vi "FTW_AppLauncher-Core_Initialize.vi"(0 "Initialization Sequence":string, 5 "FTW Actor Instance Configuration":string, 11 "error in (no error)":errorcluster) -> (4 "Actor Template-Core out":refnum<class "FTW-AppLauncher-Core.lvclass">, 6 "Event Refnums":T1, 10 "Refresh Period":dbl, 15 "error out":errorcluster)   [LabVIEW 2015, in "FTW-AppLauncher-Core.lvclass"]
uses:
  FTW-AppLauncher-Core.lvclass
  source/actor/Message/Request/FTW-Message-IncomingRequest.lvclass
  source/actor/Message/Base/FTW-Message.lvclass
  FTW-AppLauncher-Core.lvclass/FTW-AppLauncher-Core.ctl
  source/actor/Instance/FTW-ActorInstance.lvclass/FTW-ActorInstance.ctl
  source/Error/FTW-ERR-NoErrorConstant.vi
  source/JSON/FTW-JSON-Core-LibraryFilepath.vi
  source/Error/FTW-ERR-ThrowError.vi
  source/JSON/core/FTW-JSON-Core-EncodingFlags.vi
  source/Reflection/FTW-Reflection-Type.vi
  source/CodeGen/JSON Deserialize/FTW-JSON-Core-GetFlattenedValue.vi
  source/CodeGen/JSON Deserialize/FTW-JSON-Deserialize.xnode
  source/actor/Instance/FTW-ActorInstance.lvclass
  source/actor/Ether/FTW-Ether.lvclass
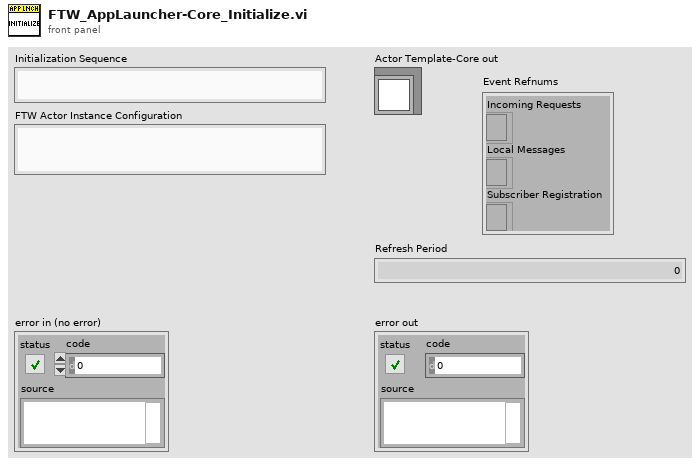
[diagram p1: front panel]
types:
  T1 = cluster{"Incoming Requests":refnum<event-registration>, "Local Messages":refnum<event-registration>, "Subscriber Registration":refnum<event-registration>}
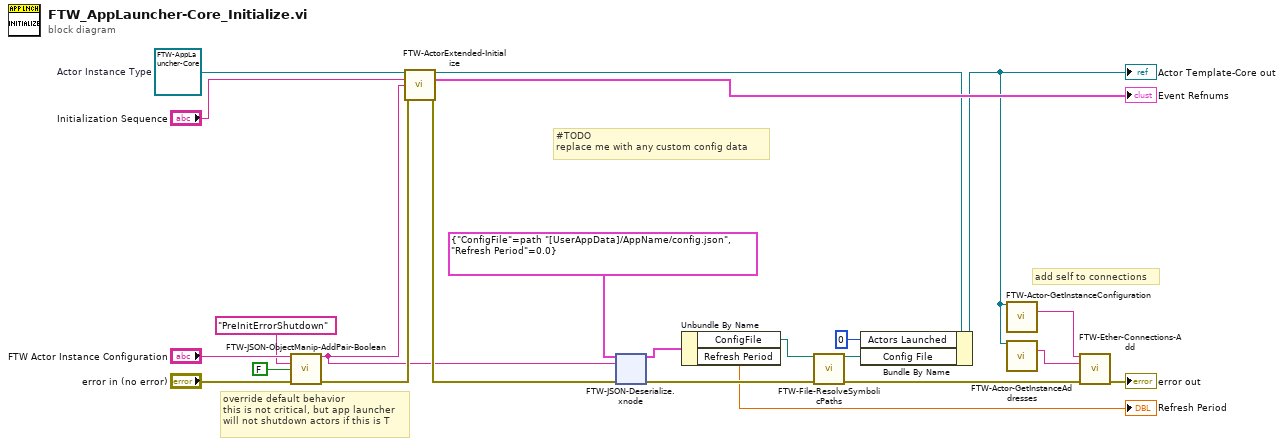
[diagram p0: block diagram]
diagram:
  w23 = refnum<class "FTW-AppLauncher-Core.lvclass"> refnum  # Actor Instance Type
  # "override default behavior\nthis is not critical, but app launcher\nwill not shutdown actors if this is T"
  # "add self to connections"
  # "#TODO\nreplace me with any custom config data"
  n1 = call "FTW-JSON-ObjectManip-AddPair-Boolean.vi"("Input JSON Object"="FTW Actor Instance Configuration", "Key"="PreInitErrorShutdown", "Value"=FALSE, "error in"="error in (no error)") -> ("Output JSON Object"=w7:string, "error out"=w9:errorcluster)  [unwired: 10 in]
  n2 = call-dynamic "FTW-ActorExtended-Initialize.vi"("FTW Actor Instance Type"=w23, "Initialization Job Sequence"="Initialization Sequence", "Actor Instance Configuration"=w7, "error in"=w9) -> ("FTW Actor Instance"=w10:refnum<class "FTW-AppLauncher-Core.lvclass">, "Event Refnums"=→"Event Refnums":T1, "error out"=w18:errorcluster)  [unwired: 9 in]
  n3 = xnode "FTW-JSON-Deserialize.xnode"("Type and Defaults"=cluster{"ConfigFile":path, "Refresh Period":dbl} {"ConfigFile"=path "[UserAppData]/AppName/config.json", "Refresh Period"=0.0}, "JSON String"=w7, "error in"=w18) -> ("Values"=w20:cluster{"ConfigFile":path, "Refresh Period":dbl}, "error out"=w22:errorcluster)
  n4 = Unbundle By Name(w20) -> ("ConfigFile"=w14:path, "Refresh Period"=→"Refresh Period":dbl)
  n5 = call "FTW-File-ResolveSymbolicPaths.vi"("Unresolved Path"=w14, "error in"=w22) -> ("Resolved Path"=w13:path, "error out"=w15:errorcluster)  [unwired: 12 in]
  n6 = Bundle By Name(cluster=w10, "Actors Launched"=0 ("Launch Step"), "Config File"=w13) -> (w4:refnum<class "FTW-AppLauncher-Core.lvclass">)
  "Actor Template-Core out" <- w4
  n7 = call "FTW-Actor-GetInstanceConfiguration.vi"("FTW Actor Instance"=w4) -> ("Identity"=w2:string)  [unwired: 12 in, 2 out]
  n8 = call "FTW-Actor-GetInstanceAddresses.vi"("FTW Actor Instance"=w4) -> ("Inbox Address"=w1:string)  [unwired: 12 in, 2 out]
  n9 = call "FTW-Ether-Connections-Add.vi"("Connection"=w2, "Address"=w1, "error in"=w15) -> ("error out"=→"error out":errorcluster)  [unwired: 12 in]
